vi "OK Button Press.vi"(8 "error in (no error)":errorcluster, 10 "Data":variant, 11 "CheckPasswordUI in":refnum<class "CheckPasswordUI.lvclass">) -> (0 "error out":errorcluster, 3 "CheckPasswordUI out":refnum<class "CheckPasswordUI.lvclass">)   [LabVIEW 2021, in "CheckPasswordUI.lvclass"]
uses:
  CheckPasswordUI.lvclass
  CheckUser.ctl
  <userlib>/John_Lib/Interfaces/InsertSubPanel/InsertSubPanel Messages/Insert SubPanel Msg/Insert SubPanel Msg.lvclass
  <vilib>/ActorFramework/Actor/Actor.lvclass
  C:/Program Files (x86)/National Instruments/LabVIEW 2021/user.lib/John_Lib/AbstractActorTemplate/AbstractActorTemplate/UIActorTop.lvclass
  C:/Program Files (x86)/National Instruments/LabVIEW 2021/vi.lib/ActorFramework/Actor/Actor.lvclass
  C:/Program Files (x86)/National Instruments/LabVIEW 2021/project/Create Actor from Template/_CheckPasswordUI/CheckPasswordUI.lvclass
  C:/Program Files (x86)/National Instruments/LabVIEW 2021/user.lib/John_Lib/Interfaces/CheckPassWord/CheckPassWord.lvclass
  C:/Program Files (x86)/National Instruments/LabVIEW 2021/user.lib/John_Lib/Interfaces/InsertSubPanel/InsertSubPanel.lvclass
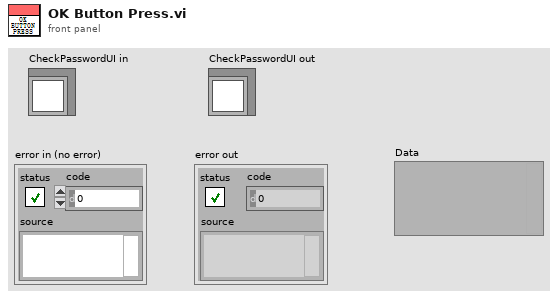
[diagram p1: front panel]
types:
  T1 = typedef "CheckPasswordUI.lvclass/CheckUser.ctl" = cluster{"UserName":string, "Password":string, "OK":bool, "Cancle":bool, "Messages":string}
  T2 = typedef "CheckPasswordUI.lvclass/DVR.ctl" = cluster{"Caller ActorQName":string, "Permission":T3, "PermissionNum":i32}
  T3 = typedef "CheckPassWord.lvlib/CheckPassWord.lvclass/Permission.ctl" = string
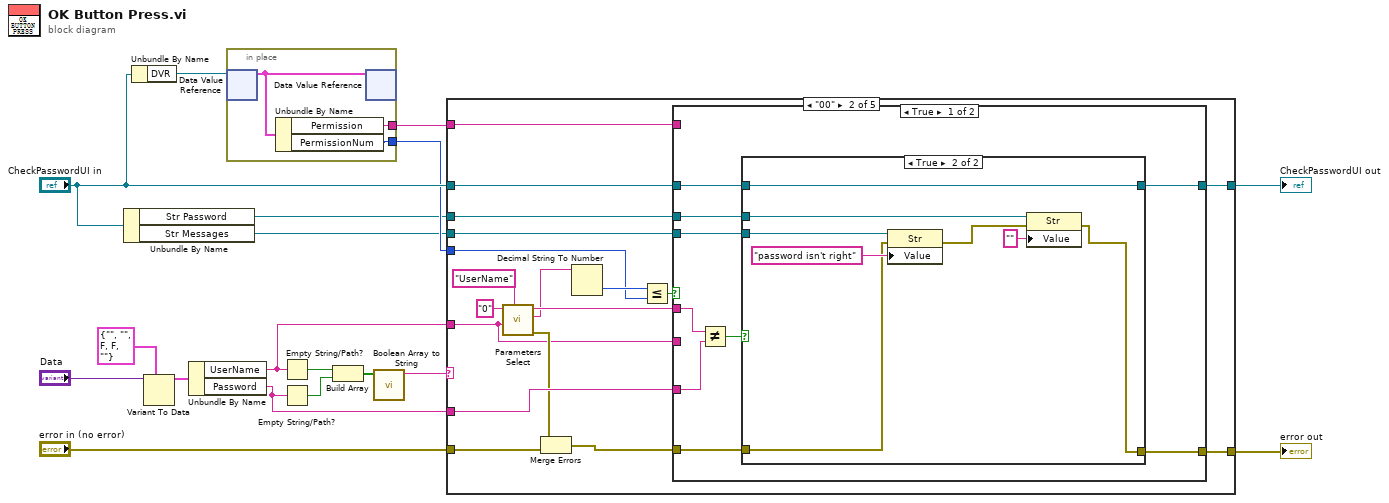
[diagram p0: block diagram]
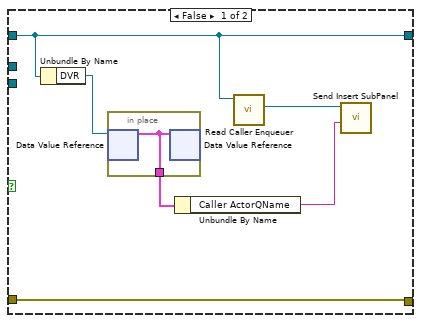
[diagram p3: hidden frame]
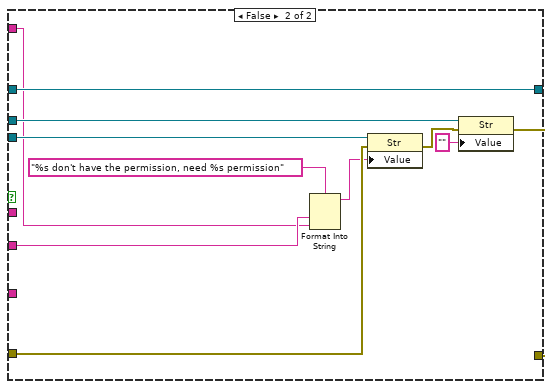
[diagram p4: hidden frame]
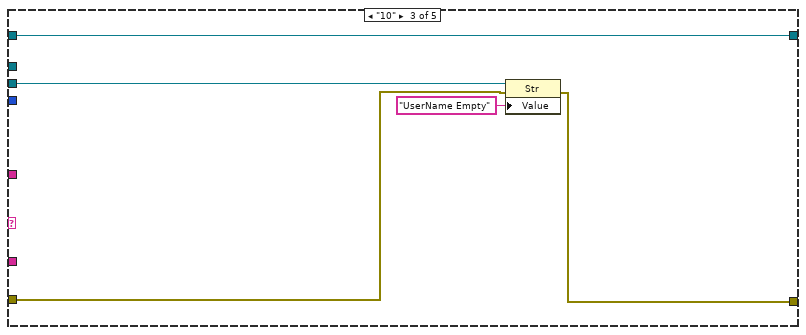
[diagram p5: hidden frame]
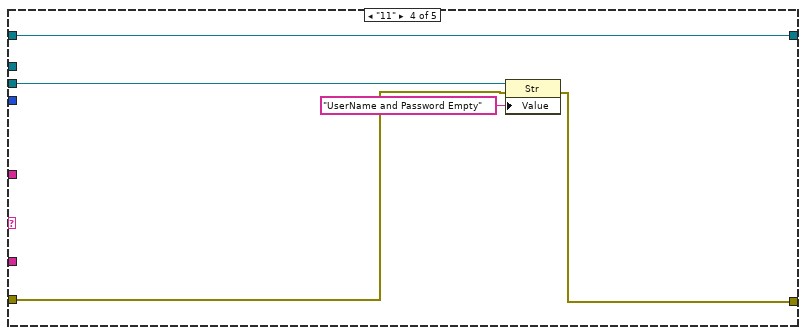
[diagram p6: hidden frame]
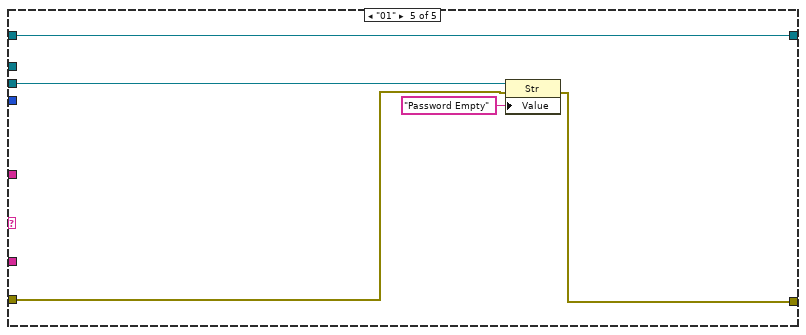
[diagram p7: hidden frame]
diagram:
  n1 = Unbundle By Name("CheckPasswordUI in") -> ("Str Password"=w2:refnum<vi>, "Str Messages"=w1:refnum<vi>)
  n2 = Unbundle By Name("CheckPasswordUI in") -> ("DVR"=w12:refnum<data-value>)
  n3 = Variant To Data(type=T1 {"UserName"="", "Password"="", "OK"=FALSE, "Cancle"=FALSE, "Messages"=""} ("CheckUser"), Variant="Data") -> (data=w13:T1)  [unwired: 1 in, 1 out]
  n4 = Unbundle By Name(w13) -> ("UserName"=w5:string, "Password"=w6:string)
  n5 = in-place {
    in-place-border: [w20] -> w3
    in-place-border: [w19] -> w4
    n6 = in-place-dvr #1(w12) -> (w21:T2)  [unwired: 1 out]
    n7 = Unbundle By Name(w21) -> ("Permission"=w19:T3, "PermissionNum"=w20:i32)
    n8 = in-place-dvr #1(w21) -> ()  [unwired: 2 out]
  }
  n9 = Empty String/Path?(string/path=w5) -> (empty?=w14:bool)
  n10 = Empty String/Path?(string/path=w6) -> (empty?=w16:bool)
  n11 = Build Array(w14, w16) -> (w15:bool[])
  n12 = call <userlib>:"Boolean Array to String.vi"("Bolean Array"=w15) -> ("Bolean String"=w7:string)  [unwired: 10 in]
  n13 = case shown="\"00\"" w7 {
    tunnel: [w23 w40 w81 w86 w91] -> w10
    tunnel: "CheckPasswordUI in" -> [w23 w39 w81 w86 w91]
    tunnel: w1 -> [_ w38 w80 w85 w90]
    tunnel: w5 -> [_ w25 _ _ _]
    tunnel: w6 -> [_ w37 _ _ _]
    tunnel: "error in (no error)" -> [w22 w33 w79 w84 w89]
    tunnel: [w22 w36 w78 w83 w88] -> w9
    tunnel: w2 -> [_ w35 _ _ _]
    tunnel: w3 -> [_ w27 _ _ _]
    tunnel: w4 -> [_ w24 _ _ _]
    frame "False", Default {
    }
    frame "00" {
      n14 = call <userlib>:"Parameters Select.vi"("Main"="UserName", "VariableName"=w25, "Sub"="0") -> ("error out"=w31:errorcluster, "Value2"=w29:string, "Value1"=w41:string)  [unwired: 4 in, 2 out]
      n15 = Merge Errors(w31, w33) -> (w32:errorcluster)
      n16 = Decimal String To Number(string=w29) -> (number=w28:i32)  [unwired: 2 in, 1 out]
      n17 = Less Or Equal?(x=w28, y=w27) -> (x <= y?=w26:bool)
      n18 = case shown="True" w26 {
        tunnel: w41 -> [w50 _]
        tunnel: [w48 w67] -> w40
        tunnel: w39 -> [w47 w67]
        tunnel: w38 -> [w46 w76]
        tunnel: w37 -> [w45 _]
        tunnel: [w44 w75] -> w36
        tunnel: w35 -> [w43 w74]
        tunnel: w32 -> [w42 w73]
        tunnel: w25 -> [_ w68]
        tunnel: w24 -> [_ w66]
        frame True {
          n19 = Not Equal?(x=w50, y=w45) -> (x != y?=w49:bool)
          n20 = case shown="True" w49 {
            tunnel: w47 -> [w54 w65]
            tunnel: [w54 w65] -> w48
            tunnel: w46 -> [_ w64]
            tunnel: w42 -> [w56 w62]
            tunnel: [w56 w59] -> w44
            tunnel: w43 -> [_ w61]
            frame False {
              n21 = Unbundle By Name(w54) -> ("DVR"=w53:refnum<data-value>)
              n22 = in-place {
                in-place-border: [w57] -> w52
                n23 = in-place-dvr #2(w53) -> (w57:T2)  [unwired: 1 out]
                n24 = in-place-dvr #2(w57) -> ()  [unwired: 2 out]
              }
              n25 = Unbundle By Name(w52) -> ("Caller ActorQName"=w51:string)
              n26 = call <vilib>:"Read Caller Enqueuer.vi"("Actor"=w54) -> ("Caller Enqueuer"=w55:refnum<class "Message Enqueuer.lvclass">)  [unwired: 10 in]
              n27 = call <userlib>:"Send Insert SubPanel.vi"("ActorQName"=w51, "Message Enqueuer"=w55) -> ()  [unwired: 8 in, 2 out]
            }
            frame True {
              n28 = property class="Str"(reference=w64, error in=w62, "Value"="password isn't right") -> (error out=w60:errorcluster)  [unwired: 1 out]
              n29 = property class="Str"(reference=w61, error in=w60, "Value"="") -> (error out=w59:errorcluster)  [unwired: 1 out]
            }
          }
        }
        frame False {
          n30 = Format Into String(format string="%s don't have the permission, need %s permission", w68, w66) -> (resulting string=w69:string)  [unwired: 2 in, 1 out]
          n31 = property class="Str"(reference=w76, error in=w73, "Value"=w69) -> (error out=w72:errorcluster)  [unwired: 1 out]
          n32 = property class="Str"(reference=w74, error in=w72, "Value"="") -> (error out=w75:errorcluster)  [unwired: 1 out]
        }
      }
    }
    frame "10" {
      n33 = property class="Str"(reference=w80, error in=w79, "Value"="UserName Empty") -> (error out=w78:errorcluster)  [unwired: 1 out]
    }
    frame "11" {
      n34 = property class="Str"(reference=w85, error in=w84, "Value"="UserName and Password Empty") -> (error out=w83:errorcluster)  [unwired: 1 out]
    }
    frame "01" {
      n35 = property class="Str"(reference=w90, error in=w89, "Value"="Password Empty") -> (error out=w88:errorcluster)  [unwired: 1 out]
    }
  }
  "error out" <- w9
  "CheckPasswordUI out" <- w10
